vi "Get Files List.vi"(7 "Folder Name":string="Tests", 8 "error in (no error)":errorcluster) -> (0 "error out":errorcluster, 3 "List":string[](array[string]))   [LabVIEW 2020, in "Settings.lvlib"]
uses:
  Settings.lvlib
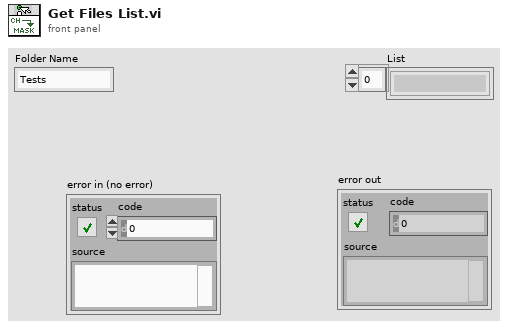
[diagram p1: front panel]
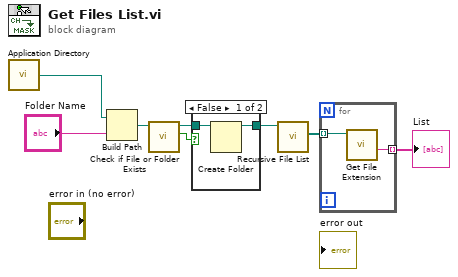
[diagram p0: block diagram]
diagram:
  n1 = call <vilib>:"Application Directory.vi"() -> ("Application Directory"=w8:path)
  n2 = Build Path(base path=w8, name or relative path="Folder Name") -> (appended path=w2:path)
  n3 = call <vilib>:"Check if File or Folder Exists.vi"("path"=w2) -> ("file or folder exists?"=w4:bool, "dup path"=w3:path)  [unwired: 8 in, 1 out]
  n4 = case shown="False" w4 {
    tunnel: w3 -> [w10 w11]
    tunnel: [w9 w11] -> w1
    frame False {
      n5 = Create Folder(path (use dialog)=w10) -> (created path=w9:path)  [unwired: 2 in, 2 out]
    }
    frame True {
    }
  }
  n6 = call <vilib>:"Recursive File List.vi"("Folder Path"=w1) -> ("All Files in Dir"=w6:path[])  [unwired: 6 in, 4 out]
  n7 = for {
    tunnel: w6 -> [w13] mode=indexing
    tunnel: [w12] -> w5 mode=indexing
    n8 = call <vilib>:"Get File Extension.vi"("file"=w13) -> ("filename without extension"=w12:string)  [unwired: 6 in, 4 out]
  }
  "List" <- w5
